vi "Hikvision 4004Hc Recorder.vi"() -> ()   [LabVIEW 2011]
uses:
  <vilib>/Platform/TimedLoop/XDataNode/timing_clust.ctl
  <vilib>/Platform/TimedLoop/XDataNode/nitl_modes.ctl
  <vilib>/Platform/TimedLoop/XDataNode/wakeup.ctl
  <vilib>/Platform/TimedLoop/XDataNode/XDataNode.xnode
  <vilib>/Platform/TimedLoop/XDataNode/XDNodeRunTimeDep.lvlib
panel:
  in  "filter":u16(ring)=14 items=["DV Video Encoder", "ffdshow video encoder", "Indeo? video 5.10 Compression Filter", "MJPEG Compressor", "Cinepak Codec by Radius", "DivX 6.9.2 Codec (2 Logical CPUs)", "Intel Indeo(R) Video R3.2", "Intel Indeo? Video 4.5", "Indeo? video 5.10", "Intel IYUV codec", "Microsoft RLE", "Microsoft Video 1", "Microsoft Windows Media Video 9", "x264vfw - H.264/MPEG-4 AVC codec", "no filter"]
  in  "Filter Names":string[](array[string])
  out "Hue":i32
  out "Saturation":i32
  in  "Contrast":i32(slide) min=0 max=127 scale=0.0..127.0
  in  "Brightness":i32(slide) min=0 max=255 scale=0.0..255.0
  out "VideoStandard":string
  out "hChannelHandle":u32
  out "返回类型 2":i32
  out "Elapsed Time (s)":dbl caption="已用时间(s)"
  out "Image":T1(plugin-control)
  in  "AVI Path":path=path "C:/Documents and Settings/pan/桌面/work/Training System 2011/Eye Traker/movie/test001.avi"
  out "返回类型":i32
  in  "停止":bool
  out "获取数据循环持续时间":u64
  in  "record":bool
  out "错误输出":errorcluster
  out "数据处理循环持续时间":u64
  out "ChannelOpen":u32 format="%x"
  out "GetTotalChannels":i32
  out "InitDSPs":i32
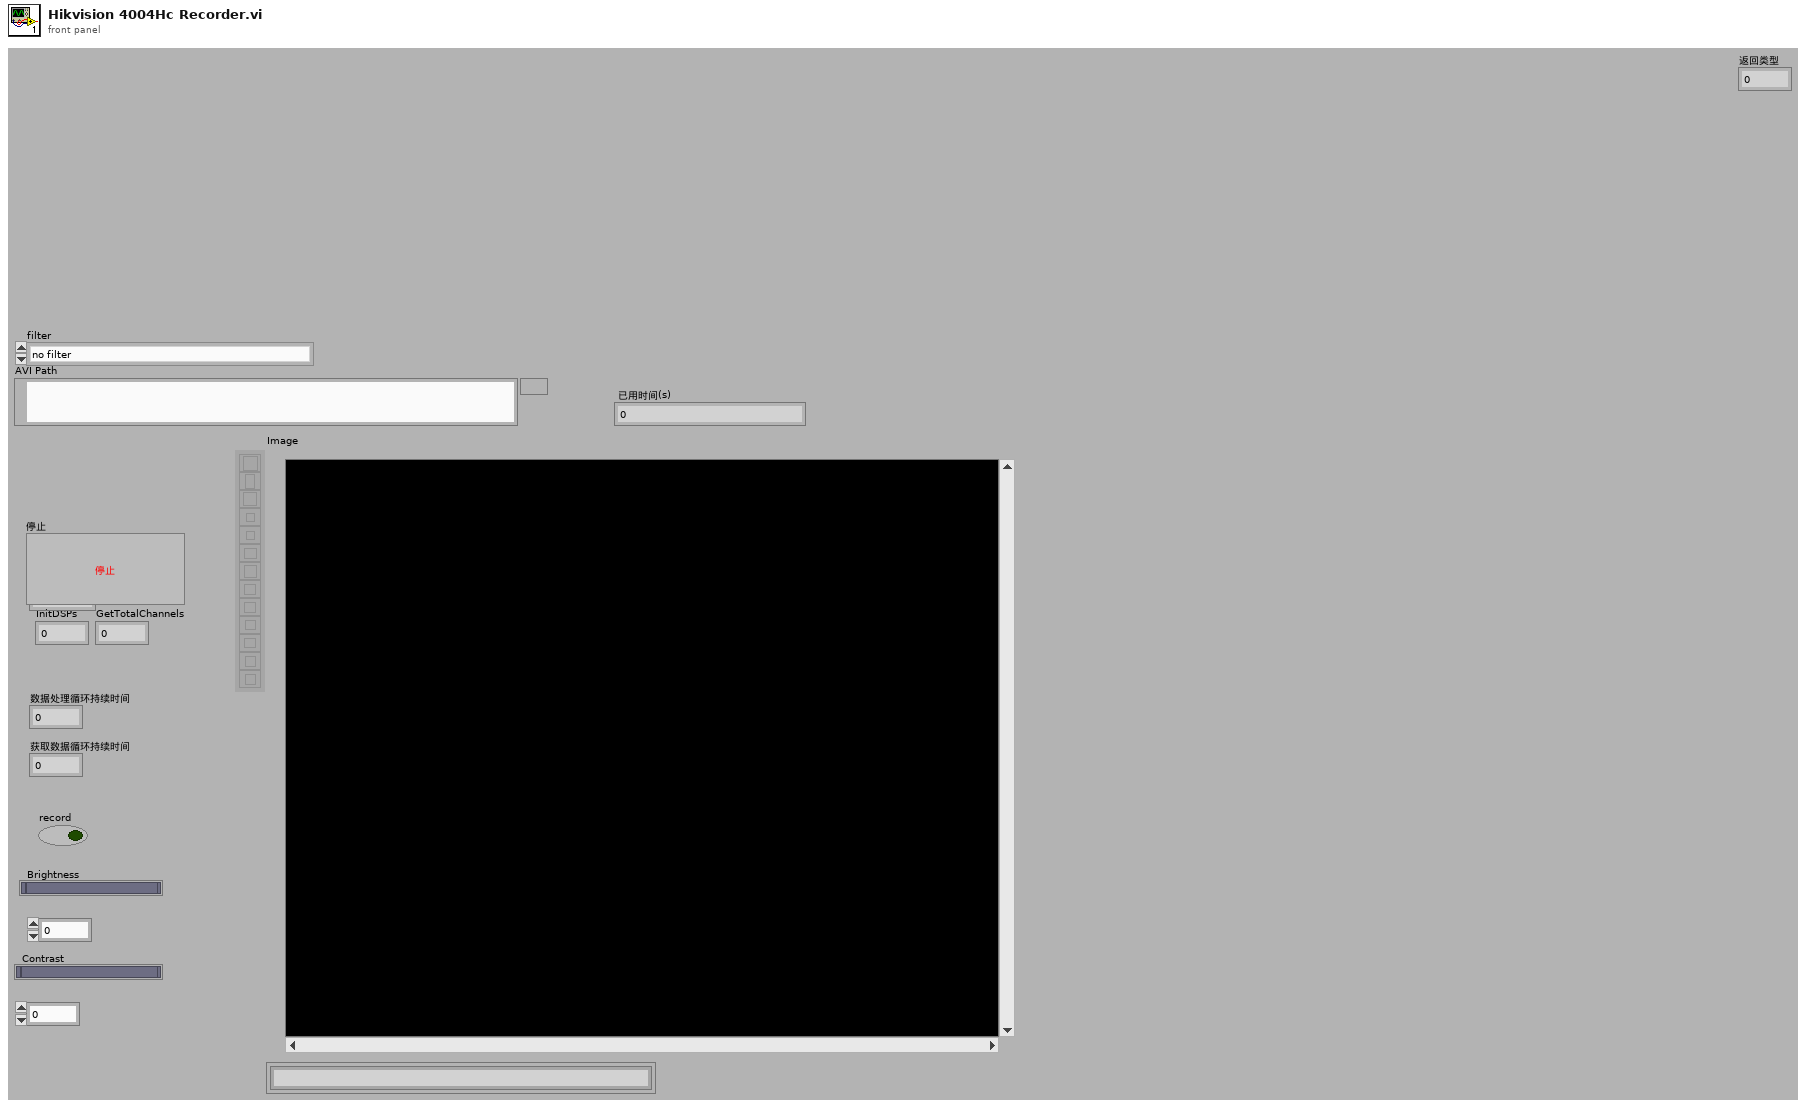
[diagram p1: front panel]
types:
  T1 = typedef "IMAQ Image.ctl" = refnum<image>
  T2 = typedef "XDNodeRunTimeDep.lvlib/timing_clust.ctl" = cluster{"Expected End [f-1]":u64, "Actual End [f-1]":u64, "Finished Late? [f-1]":bool, "Expected End [i-1]":u64, "Actual End [i-1]":u64, "Finished Late? [i-1]":bool, "Expected Start [i]":u64, "Actual Start [i]":u64, "Expected Start [f]":u64, "Actual Start [f]":u64, "Source Name":string, "Structure Name":string, "Period":i64, "Deadline":i64, "Offset":i64, "Start":i64, "Priority":i32, "Timeout":i32, "Mode":T3, "Wakeup Reason":T4, "Error":errorcluster, "Source Type":string, "Secondary Source Type":string, "Global End Time":u64, "Global Start Time":u64, "Frame Duration":u64, "Iteration Duration":u64, "Assigned CPU":i32, "I/O Scan Engine Mode":u32}
  T3 = typedef "XDNodeRunTimeDep.lvlib/nitl_modes.ctl" = enum32{"No Change", "Process missed periods, maintain original phase", "Discard missed periods, maintain original phase", "Process missed periods, ignore original phase", "Discard missed periods, ignore original phase"}
  T4 = typedef "XDNodeRunTimeDep.lvlib/wakeup.ctl" = enum32{"Normal", "Aborted", "Asynchronous wakeup", "Timing source error", "Timed loop error", "Timeout"}
  T5 = typedef "Image Type" = u32
  T6 = typedef "AviRefnum.ctl" = refnum<k1>
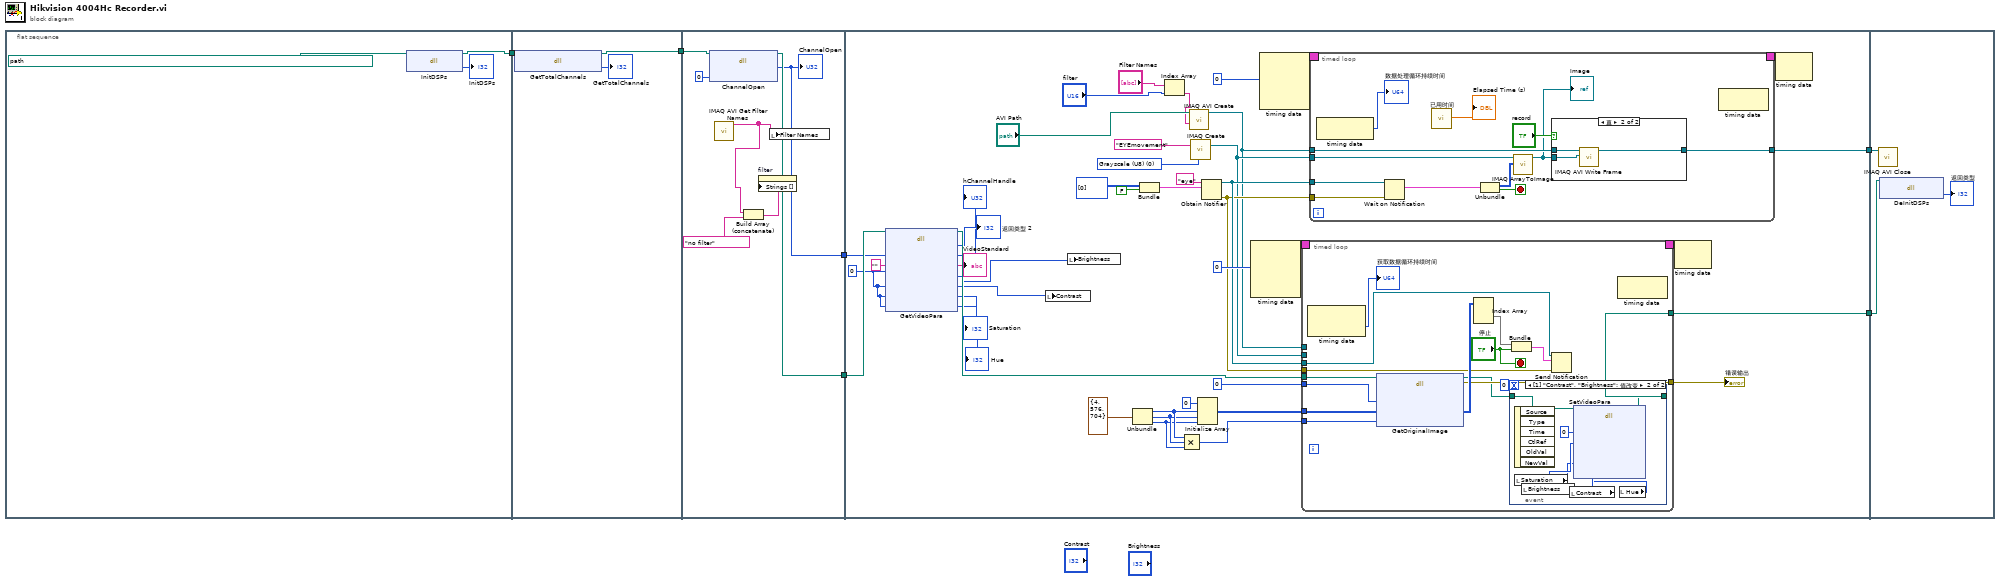
[diagram p0: block diagram]
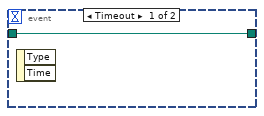
[diagram p3: hidden frame]
diagram:
  n1 = flat-sequence {
    tunnel: [w7] -> w5
    tunnel: w5 -> [w11]
    tunnel: [w10] -> w4
    tunnel: w4 -> [w18]
    tunnel: [w17] -> w3
    tunnel: [w16] -> w1
    tunnel: [w36] -> w6
    tunnel: w3 -> [w34]
    tunnel: [w35] -> w2
    tunnel: w1 -> [w32]
    tunnel: w6 -> [w117]
    tunnel: w2 -> [w116]
    frame #0 {
      n2 = dll-call lib="PTH1labs C\nProgram Files\tHikvision+DS-4000系列板卡SDK and Demo Version 5.1SDKcard sdk\nDs40xxSDK.dll" fn="InitDSPs"(path in=path "C:/Program Files/Hikvision/DS-4000系列板卡SDK and Demo Version 5.1/SDK/card sdk/Ds40xxSDK.dll" ("路径输入")) -> (path out=w7:path, "返回类型"=→"InitDSPs":i32)  [unwired: 2 in, 1 out]
    }
    frame #1 {
      n3 = dll-call lib="PTH1labs C\nProgram Files\tHikvision+DS-4000系列板卡SDK and Demo Version 5.1SDKcard sdk\nDs40xxSDK.dll" fn="GetTotalChannels"(path in=w11) -> (path out=w10:path, "返回类型"=→"GetTotalChannels":i32)  [unwired: 2 in, 1 out]
    }
    frame #2 {
      n4 = dll-call lib="PTH1labs C\nProgram Files\tHikvision+DS-4000系列板卡SDK and Demo Version 5.1SDKcard sdk\nDs40xxSDK.dll" fn="ChannelOpen"(path in=w18, "ChannelNum"=0) -> (path out=w17:path, "返回类型"=w16:u32)  [unwired: 3 in, 1 out]
      "ChannelOpen" <- w16
      n5 = call "IMAQ AVI Get Filter Names"() -> ("Filter Names"=w15:string[])  [unwired: 1 in, 10 out]
      n6 = Build Array (concatenate)(w15, "no filter") -> (w13:string[])
      n7 = property on="filter" class="Ring (严格)"("Strings []"=w13) -> ()  [unwired: 2 in, 2 out]
      n8 = local write "Filter Names"(w15) -> ()
    }
    frame #3 {
      w30 = 0 ("Brightness")
      w41 = T5 0 items=["Grayscale (U8)", "Grayscale (I16)", "Grayscale (SGL)", "Complex (CSG)", "RGB (U32)", "HSL (U32)", "RGB (U64)", "Grayscale (U16)"] ("Image Type")
      n9 = dll-call lib="PTH1babs C\nProgram Files\tHikvision+DS-4000系列板卡SDK and Demo Version 5.1Bin\nDs40xxSDK.dll" fn="GetVideoPara"(path in=w34, "hChannelHandle"=w32, "VideoStandard"="", "Brightness"=w30, "Contrast"=w30, "Saturation"=w30, "Hue"=w30) -> (path out=w33:path, "返回类型"=→"返回类型 2":i32, "hChannelHandle"=→"hChannelHandle":u32, "VideoStandard"=→"VideoStandard":string, "Brightness"=w23:i32, "Contrast"=w24:i32, "Saturation"=→"Saturation":i32, "Hue"=→"Hue":i32)  [unwired: 2 in, 1 out]
      n10 = local write "Contrast"(w24) -> ()
      n11 = local write "Brightness"(w23) -> ()
      n12 = Unbundle(cluster{"元素":i32, "元素 2":i32, "元素 3":i32} {"元素"=4, "元素 2"=576, "元素 3"=704}) -> ("元素"=w56:i32, "元素 2"=w55:i32, "元素 3"=w54:i32)
      n13 = Bundle("子数组"=u8[][] [[0]], FALSE) -> (w44:cluster{"子数组":u8[][], bool})  [unwired: 1 out]
      n14 = Index Array(array="Filter Names", index="filter") -> (element=w22:string)
      n15 = Compound Arithmetic op=MULTIPLY(w56, w55, w54) -> (w58:i32)
      n16 = call "IMAQ AVI Create"("Compression Filter"=w22, "AVI Path"="AVI Path") -> ("Avi Refnum"=w37:T6)  [unwired: 5 in, 4 out]
      n17 = call "IMAQ Create"("Image Name"="EYEmovement", "Image Type"=w41) -> ("New Image"=w38:T1)  [unwired: 2 in, 2 out]
      n18 = Initialize Array(u8 0 ("元素"), w56, w55, w54) -> (w52:u8[][][])
      n19 = Obtain Notifier(name (unnamed)="eye" ("名称（未命名）"), notification data type=w44) -> (notifier out=w47:refnum<notifier>, error out=w46:errorcluster)  [unwired: 2 in, 1 out]
      n20 = node-c288(i64 0 ("周期")) -> (w60:T2)  [unwired: 3 out]
      n21 = node-c288(i64 0 ("周期")) -> (w49:T2)  [unwired: 3 out]
      n22 = timed-loop {
        tunnel: w52 -> [w98]
        tunnel: w58 -> [w100]
        tunnel: u32 0 ("hChannelHandle") -> [w99]
        timing: w60 -> [_]
        timing-out: [_] -> w59
        tunnel: [w95] -> w51
        tunnel: w47 -> [w94]
        tunnel: w46 -> [w93]
        tunnel: w37 -> [_]
        tunnel: w38 -> [_]
        tunnel: w33 -> [w89]
        tunnel: [w86] -> w35
        stop <- "停止" stop-if-true
        n23 = node-c288() -> (→"获取数据循环持续时间":i64)  [unwired: 2 out]
        n24 = dll-call lib="PTH1labs C\nProgram Files\tHikvision+DS-4000系列板卡SDK and Demo Version 5.1SDKcard sdk\nDs40xxSDK.dll" fn="GetOriginalImage"(path in=w89, "hChannelHandle"=w99, "ImageBuf"=w98, "Size"=w100) -> (path out=w87:path, error out=w95:errorcluster, "ImageBuf"=w96:u8[][][])  [unwired: 3 in, 2 out]
        n25 = Index Array(array=w96) -> (element=w91:u8[][])  [unwired: 3 in]
        n26 = event shown="[1] \"Contrast\", \"Brightness\": 值改变" {
          selector: _ -> [_ _]
          dyn-events: _ -> [_ _]
          timeout: 0 -> [_ _]
          tunnel: w87 -> [w101 w108]
          tunnel: [w101 w107] -> w86
          event Timeout {
            n27 = event-data() -> ()  [unwired: 3 out]
          }
          event "Contrast", "Brightness": Value Change {
            n28 = event-data() -> ()  [unwired: 7 out]
            n29 = local read "Saturation"() -> (w104:i32)
            n30 = local read "Brightness"() -> (w106:i32)
            n31 = local read "Contrast"() -> (w105:i32)
            n32 = local read "Hue"() -> (w103:i32)
            n33 = dll-call lib="PTH1babs C\nProgram Files\tHikvision+DS-4000系列板卡SDK and Demo Version 5.1Bin\nDs40xxSDK.dll" fn="SetVideoPara"(path in=w108, "hChannelHandle"=u32 0, "Brightness"=w106, "Contrast"=w105, "Saturation"=w104, "Hue"=w103) -> (path out=w107:path)  [unwired: 7 in, 2 out]
          }
        }
        n34 = Bundle("ImageBuf"=w91, "停止"="停止") -> (w90:cluster{"ImageBuf":u8[][], "停止":bool})  [unwired: 1 out]
        n35 = Send Notification(notification=w90, notifier=w94, error in (no error)=w93) -> ()  [unwired: 2 out]
        n36 = node-c288() -> ()  [unwired: 2 out]
      }
      "错误输出" <- w51
      n37 = timed-loop {
        timing: w49 -> [_]
        timing-out: [_] -> w48
        tunnel: w47 -> [w73]
        tunnel: w46 -> [w72]
        tunnel: w38 -> [w65]
        tunnel: w37 -> [w69]
        tunnel: [w68] -> w36
        stop <- w70 stop-if-true
        n38 = node-c288() -> (→"数据处理循环持续时间":i64)  [unwired: 1 out]
        n39 = Wait on Notification(notifier=w73, error in (no error)=w72) -> (notification=w71:cluster{"子数组":u8[][], bool})  [unwired: 5 out]
        n40 = call "已用时间"() -> ("Elapsed Time (s)"=→"Elapsed Time (s)":dbl)  [unwired: 5 in, 14 out]
        n41 = Unbundle(w71) -> ("子数组"=w66:u8[][], w70:bool)
        n42 = call "IMAQ ArrayToImage"("Image Pixels (U8)"=w66, "Image"=w65) -> ("Image Out"=w64:T1)  [unwired: 4 in, 5 out]
        "Image" <- w64
        n43 = case shown="真" "record" {
          tunnel: w69 -> [w75 w78]
          tunnel: [w75 w77] -> w68
          tunnel: w64 -> [_ w76]
          frame False {
          }
          frame True {
            n44 = call "IMAQ AVI Write Frame"("Image"=w76, "Avi Refnum"=w78) -> ("Avi Refnum (duplicate)"=w77:T6)  [unwired: 2 in, 7 out]
          }
        }
        n45 = node-c288() -> ()  [unwired: 2 out]
      }
      n46 = node-c288(w59) -> ()  [unwired: 1 out]
      n47 = node-c288(w48) -> ()  [unwired: 1 out]
    }
    frame #4 {
      n48 = call "IMAQ AVI Close"("Avi Refnum"=w117) -> ()  [unwired: 1 in, 10 out]
      n49 = dll-call lib="PTH1labs C\nProgram Files\tHikvision+DS-4000系列板卡SDK and Demo Version 5.1SDKcard sdk\nDs40xxSDK.dll" fn="DeInitDSPs"(path in=w116) -> ("返回类型"=→"返回类型":i32)  [unwired: 2 in, 2 out]
    }
  }
